vi "Climb_Globals.vi"() -> ()   [LabVIEW 2019]
uses:
  Subsystems/Climb/Climb_Cluster.ctl
  Subsystems/Climb/Climb_States.ctl
panel:
  in  "Climb_Transverse":string="Climb_Transverse"
  in  "Climb_Elevator_Left":string="Climb_Elevator_Left"
  in  "Climb_Elevator_Right":string="Climb_Elevator_Right"
  in  "Climb_Pivot":string="Climb_Pivot"
  in  "Climb_Execute_Notifier":refnum<notifier>
  in  "Climb_Set_Notifier":refnum<notifier>
  in  "Climb_Execute_Ref":string="Climb_Execute_Ref"
  in  "Climb_Set_Ref":string="Climb_Set_Ref"
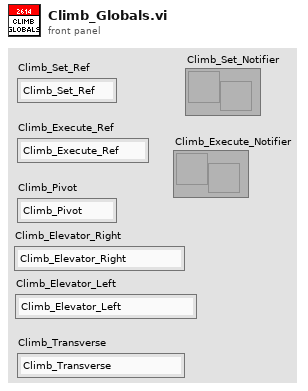
[diagram p1: front panel]
diagram:
